vi "Set Tree Symbols Based on Other.vi"(8 "error in (no error)":errorcluster, 9 "Numeric":i32, 10 "Tag":string, 11 "TreeControl in":refnum<vi>) -> (0 "error out":errorcluster)   [LabVIEW 2025, in "Protection and Counter Addon System Explorer.lvlib"]
uses:
  Protection and Counter Addon System Explorer.lvlib
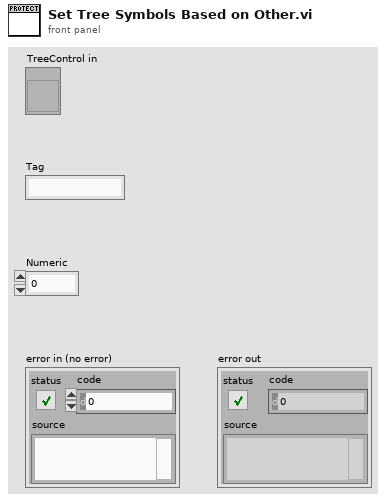
[diagram p1: front panel]
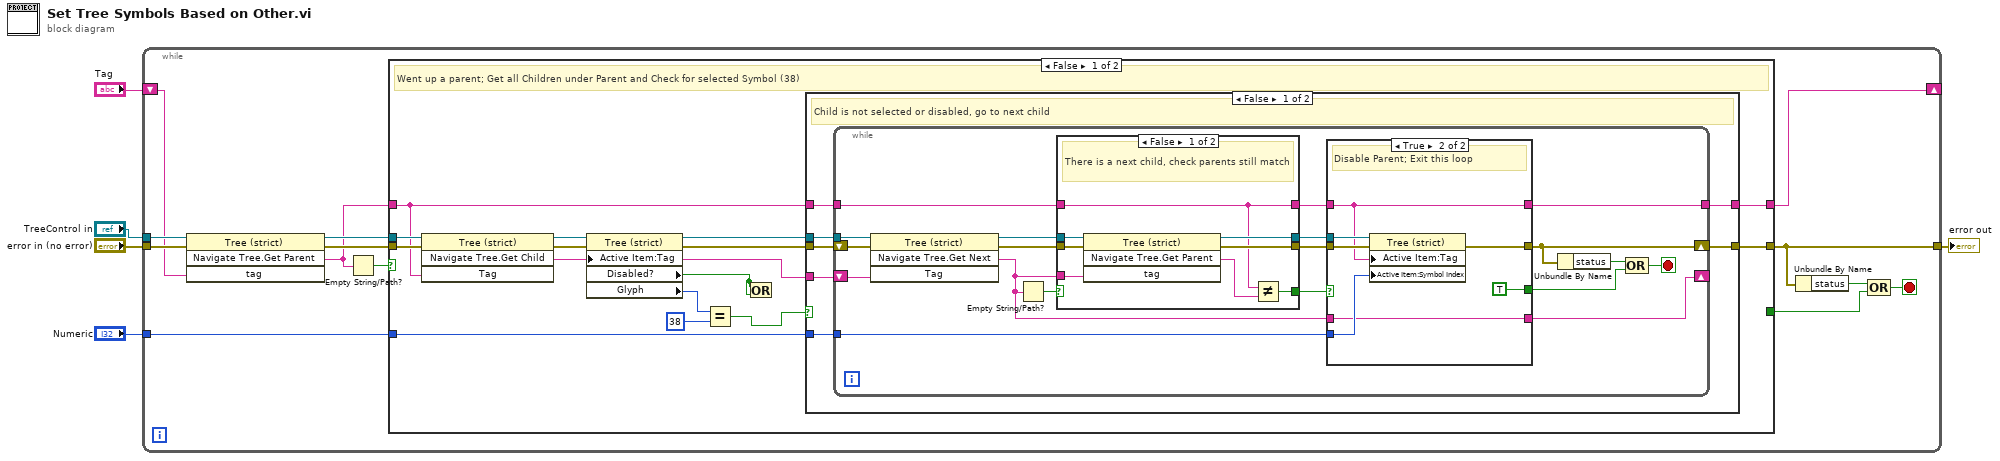
[diagram p0: block diagram]
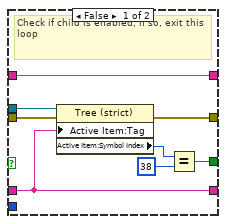
[diagram p3: hidden frame]
diagram:
  n1 = while {
    tunnel: [w9] -> w1
    tunnel: "error in (no error)" -> [w18]
    tunnel: "TreeControl in" -> [w17]
    shift-right: [w12] -> _
    shift-left: "Tag" -> [w11]
    tunnel: "Numeric" -> [w10]
    stop <- w7 stop-if-true
    n2 = invoke on="Invoke Node" class="Tree (strict)" method="Navigate Tree.Get Parent"(reference=w17, error in=w18, "tag"=w11) -> (reference out=w15:refnum<vi>, error out=w16:errorcluster, "Navigate Tree:Get Parent"=w14:string)  [unwired: 1 in, 1 out]
    n3 = Empty String/Path?(string/path=w14) -> (empty?=w13:bool)
    n4 = case shown="False" w13 {
      selector: w13 -> [_ w89]
      tunnel: w10 -> [w33 _]
      tunnel: [w32 w91] -> w9
      tunnel: w16 -> [w31 w91]
      tunnel: w15 -> [w30 _]
      tunnel: w14 -> [w25 w90]
      tunnel: [w23 w90] -> w12
      tunnel: [_ w89] -> w6
      frame False {
        # "Went up a parent; Get all Children under Parent and Check for selected Symbol (38)"
        n5 = invoke on="Invoke Node" class="Tree (strict)" method="Navigate Tree.Get Child"(reference=w30, error in=w31, "Tag"=w25) -> (reference out=w29:refnum<vi>, error out=w27:errorcluster, "Navigate Tree:Get Child"=w21:string)  [unwired: 1 in, 1 out]
        n6 = property class="Tree (strict)"(reference=w29, error in=w27, "Active Item:Tag"=w21) -> (reference out=w28:refnum<vi>, error out=w26:errorcluster, "Disabled?"=w19:bool, "Glyph"=w22:i32)
        n7 = Equal?(x=w22, y=38 ("Active Item:Symbol Index")) -> (x = y?=w20:bool)
        n8 = Or(x=w19, y=w19) -> ()  [unwired: 1 out]
        n9 = case shown="False" w20 {
          tunnel: w33 -> [w40 _]
          tunnel: [w39 w88] -> w32
          tunnel: w28 -> [w38 _]
          tunnel: w26 -> [w37 w88]
          tunnel: w21 -> [w36 _]
          tunnel: w25 -> [w35 w87]
          tunnel: [w34 w87] -> w23
          frame False {
            # "Child is not selected or disabled, go to next child"
            n10 = while {
              tunnel: w40 -> [w59]
              tunnel: w38 -> [w56]
              shift-right: [w46] -> w39
              shift-left: w37 -> [w58]
              shift-right: [w41] -> _
              shift-left: w36 -> [w57]
              tunnel: w35 -> [w47]
              tunnel: [w42] -> w34
              stop <- w44 stop-if-true
              n11 = invoke on="Invoke Node" class="Tree (strict)" method="Navigate Tree.Get Next"(reference=w56, error in=w58, "Tag"=w57) -> (reference out=w55:refnum<vi>, error out=w53:errorcluster, "Navigate Tree:Get Next Item"=w48:string)  [unwired: 1 in, 1 out]
              n12 = Empty String/Path?(string/path=w48) -> (empty?=w50:bool)
              n13 = case shown="False" w50 {
                selector: w50 -> [_ w71]
                tunnel: w55 -> [w67 w69]
                tunnel: [w66 w69] -> w54
                tunnel: w53 -> [w65 w70]
                tunnel: [w64 w70] -> w52
                tunnel: [w62 w71] -> w51
                tunnel: w47 -> [w60 w68]
                tunnel: w48 -> [w61 _]
                tunnel: [w60 w68] -> w49
                frame False {
                  # "There is a next child, check parents still match"
                  n14 = invoke on="Invoke Node" class="Tree (strict)" method="Navigate Tree.Get Parent"(reference=w67, error in=w65, "tag"=w61) -> (reference out=w66:refnum<vi>, error out=w64:errorcluster, "Navigate Tree:Get Parent"=w63:string)  [unwired: 1 in, 1 out]
                  n15 = Not Equal?(x=w60, y=w63) -> (x != y?=w62:bool)
                }
                frame True {
                }
              }
              n16 = case shown="True" w51 {
                tunnel: w59 -> [_ w82]
                tunnel: w52 -> [w79 w84]
                tunnel: [w74 w85] -> w46
                tunnel: w54 -> [w78 w83]
                tunnel: w48 -> [w72 w80]
                tunnel: [w75 TRUE] -> w43
                tunnel: w49 -> [w73 w81]
                tunnel: [w73 w81] -> w42
                tunnel: [w72 w80] -> w41
                frame False {
                  # "Check if child is enabled, if so, exit this loop"
                  n17 = property class="Tree (strict)"(reference=w78, error in=w79, "Active Item:Tag"=w72) -> (error out=w74:errorcluster, "Active Item:Symbol Index"=w76:i32)  [unwired: 1 out]
                  n18 = Equal?(x=w76, y=38 ("Active Item:Symbol Index")) -> (x = y?=w75:bool)
                }
                frame True {
                  # "Disable Parent; Exit this loop"
                  n19 = property class="Tree (strict)"(reference=w83, error in=w84, "Active Item:Tag"=w81, "Active Item:Symbol Index"=w82) -> (error out=w85:errorcluster)  [unwired: 1 out]
                }
              }
              n20 = Unbundle By Name(w46) -> ("status"=w45:bool)
              n21 = Compound Arithmetic op=OR(w45, w43) -> (w44:bool)
            }
          }
          frame True {
            # "Item is Disable or Enabled so skip this child."
          }
        }
      }
      frame True {
        # "Empty; No more parents to go"
      }
    }
    n22 = Unbundle By Name(w9) -> ("status"=w8:bool)
    n23 = Compound Arithmetic op=OR(w8, w6) -> (w7:bool)
  }
  "error out" <- w1
